vi "Write Control Values to FileProvider_ini.vi"(7 "Instrument CFGs":string[](array[string]), 8 "Series CFG Value":string, 9 "Series CFG Path Value":path, 10 "Virt Instrs CFG Value":string, 11 "Virt Instrs CFG Path Value":path) -> (0 "error out":errorcluster)   [LabVIEW 2024, in "File Provider.lvlib" / "File Provider.lvclass"]
uses:
  File Provider.lvclass
  File Provider.lvclass/File Provider.ctl
  <vilib>/Utility/config.llb/NI_LVConfig.lvlib
  <vilib>/Utility/config.llb/Write Key (String).vi
  <vilib>/Utility/config.llb/Write Key (Path).vi
  <vilib>/Utility/config.llb/Write Key (I32).vi
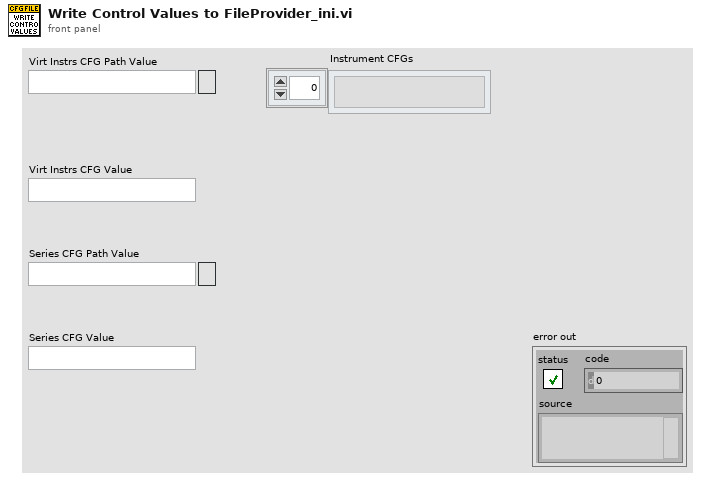
[diagram p1: front panel]
types:
  T1 = typedef "NI_LVConfig.lvlib/Config Data RefNum.ctl" = refnum<k1>
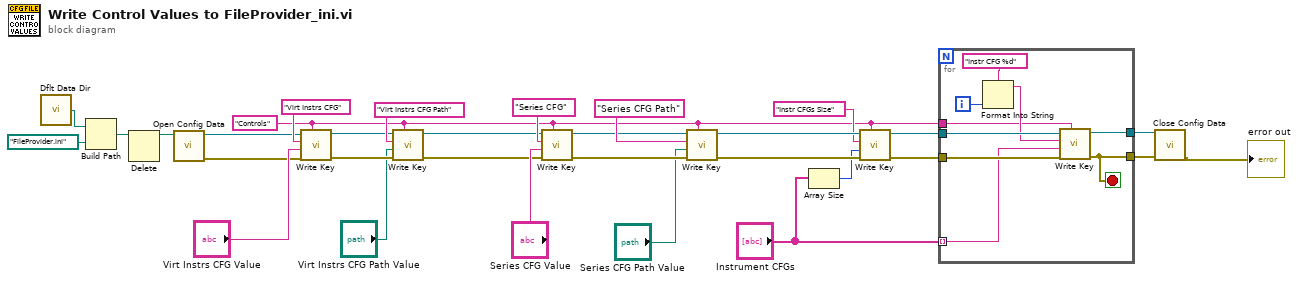
[diagram p0: block diagram]
diagram:
  w1 = "Controls" ("section")
  n1 = call <vilib>:"Dflt Data Dir.vi"() -> ("App:Default Data Directory"=w29:path)
  n2 = Build Path(base path=w29, name or relative path=path "FileProvider.ini" ("default name")) -> (appended path=w31:path)
  n3 = Delete(path (use dialog)=w31) -> (deleted path=w30:path)  [unwired: 4 in, 2 out]
  n4 = call <vilib>:"Open Config Data.vi"("configuration file path"=w30) -> ("error out"=w14:errorcluster, "refnum"=w13:T1)  [unwired: 2 in, 7 out]
  n5 = call-poly <vilib>:"Write Key.vi"("section"=w1, "error in (no error)"=w14, "value"="Virt Instrs CFG Value", "key"="Virt Instrs CFG", "refnum"=w13) -> ("error out"=w18:errorcluster, "refnum out"=w24:T1)  [unwired: 4 in, 1 out]
  n6 = call-poly <vilib>:"Write Key.vi"("section"=w1, "error in (no error)"=w18, "value"="Virt Instrs CFG Path Value", "key"="Virt Instrs CFG Path", "refnum"=w24) -> ("error out"=w17:errorcluster, "refnum out"=w22:T1)  [unwired: 4 in, 1 out]
  n7 = call-poly <vilib>:"Write Key.vi"("section"=w1, "error in (no error)"=w17, "value"="Series CFG Value", "key"="Series CFG", "refnum"=w22) -> ("error out"=w16:errorcluster, "refnum out"=w19:T1)  [unwired: 4 in, 1 out]
  n8 = call-poly <vilib>:"Write Key.vi"("section"=w1, "error in (no error)"=w16, "value"="Series CFG Path Value", "key"="Series CFG Path", "refnum"=w19) -> ("error out"=w12:errorcluster, "refnum out"=w6:T1)  [unwired: 4 in, 1 out]
  n9 = Array Size(array="Instrument CFGs") -> (size(s)=w2:i32)
  n10 = call-poly <vilib>:"Write Key.vi"("section"=w1, "error in (no error)"=w12, "value"=w2, "key"="Instr CFGs Size" ("format string"), "refnum"=w6) -> ("error out"=w7:errorcluster, "refnum out"=w5:T1)  [unwired: 4 in, 1 out]
  n11 = for {
    tunnel: w7 -> [w40]
    tunnel: w5 -> [w39]
    tunnel: "Instrument CFGs" -> [w35] mode=indexing
    tunnel: w1 -> [w34]
    tunnel: [w33] -> w11
    tunnel: [w32] -> w10
    i -> [w38]
    stop <- w33 stop-if-true
    n12 = Format Into String(format string="Instr CFG %d", w38) -> (resulting string=w36:string)  [unwired: 2 in, 1 out]
    n13 = call-poly <vilib>:"Write Key.vi"("section"=w34, "error in (no error)"=w40, "value"=w35, "key"=w36, "refnum"=w39) -> ("error out"=w33:errorcluster, "refnum out"=w32:T1)  [unwired: 4 in, 1 out]
  }
  n14 = call <vilib>:"Close Config Data.vi"("error in (no error)"=w11, "refnum"=w10) -> ("error out"=→"error out":errorcluster)  [unwired: 1 in, 8 out]
